vi "Execute Msg Or Recurse.vi"(7 "Actor in":refnum<class "Actor.lvclass">, 10 "Msg":refnum<class "Msg.lvclass">) -> (0 "Error out":errorcluster, 2 "Msg Output":refnum<class "Msg Output.lvclass">, 5 "Actor out":refnum<class "Actor.lvclass">)   [LabVIEW 2025, in "jettl.lvlib"]
uses:
  jettl.lvlib
  Msg/Msg.lvclass
  Actor/Actor.lvclass
  Msg Output/Msg Output.lvclass
  Core Actor/Core Actor.lvlib
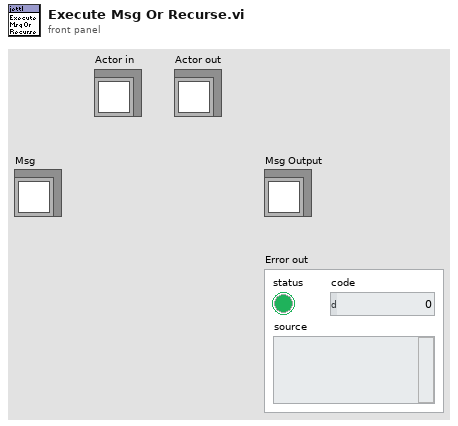
[diagram p1: front panel]
types:
  T1 = typedef "jettl.lvlib/Msg Set.ctl" = set{refnum<class "Msg.lvclass">}
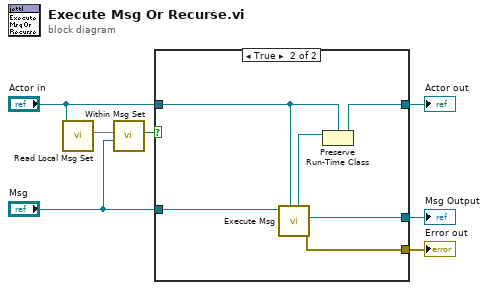
[diagram p0: block diagram]
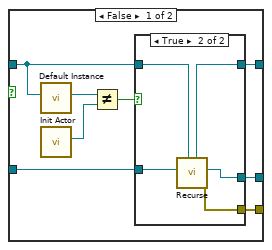
[diagram p2: hidden frame]
diagram:
  n1 = call-dynamic "Read Local Msg Set.vi"("Actor in"="Actor in") -> ("Local Msg Set"=w4:T1)  [unwired: 10 in]
  n2 = call "Within Msg Set.vi"("Msg"="Msg", "Msg Set"=w4) -> ("Within Msg Set"=w7:bool)  [unwired: 9 in]
  n3 = case shown="True" w7 {
    tunnel: "Actor in" -> [w9 w25]
    tunnel: [w13 w24] -> w2
    tunnel: "Msg" -> [w15 w27]
    tunnel: [w14 w23] -> w5
    tunnel: [w12 w22] -> w1
    frame False {
      n4 = call "Default Instance.vi"("Instance"=w9) -> ("Default Instance"=w11:refnum<class "Actor.lvclass">)  [unwired: 10 in]
      n5 = call "Init Actor.vi"() -> ("Actor"=w10:refnum<class "Actor.lvclass">)  [unwired: 11 in]
      n6 = Not Equal?(x=w11, y=w10) -> (x != y?=w8:bool)
      n7 = case shown="True" w8 {
        tunnel: w15 -> [_ w19]
        tunnel: [_ w18] -> w14
        tunnel: w9 -> [w16 w21]
        tunnel: [w16 w20] -> w13
        tunnel: [_ w17] -> w12
        frame False {
          # "This is the core, do nothing."
        }
        frame True {
          n8 = call "Recurse.vi"("Actor in"=w21, "Msg"=w19) -> ("Error out"=w18:errorcluster, "Msg Output"=w17:refnum<class "Msg Output.lvclass">, "Actor out"=w20:refnum<class "Actor.lvclass">)  [unwired: 7 in]
        }
      }
    }
    frame True {
      n9 = call-dynamic "Execute Msg.vi"("Actor in"=w25, "Msg in"=w27) -> ("Error out"=w23:errorcluster, "Msg Output"=w22:refnum<class "Msg Output.lvclass">, "Actor out"=w26:refnum<class "Actor.lvclass">)  [unwired: 7 in]
      n10 = Preserve Run-Time Class(object in=w26, 2:w25) -> (object out=w24:refnum<class "Actor.lvclass">)  [unwired: 1 in, 1 out]
    }
  }
  "Error out" <- w5
  "Actor out" <- w2
  "Msg Output" <- w1
